vi "Decoratorn2_Main.vi"() -> ()   [LabVIEW 2020]
uses:
  Circle_class/Circle.lvclass
  C:/Projects/DesignPatterns/Decorator2/Object_interface/Object.lvclass
  HappyDecorator_class/HappyDecorator.lvclass
panel:
  in  "Add Decoration?":bool
  out "2D Picture":picture
  # "Run it first without \"Add Decoration?\"\nAnd then with :-)"
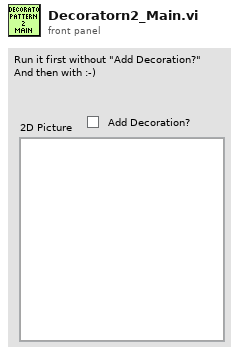
[diagram p1: front panel]
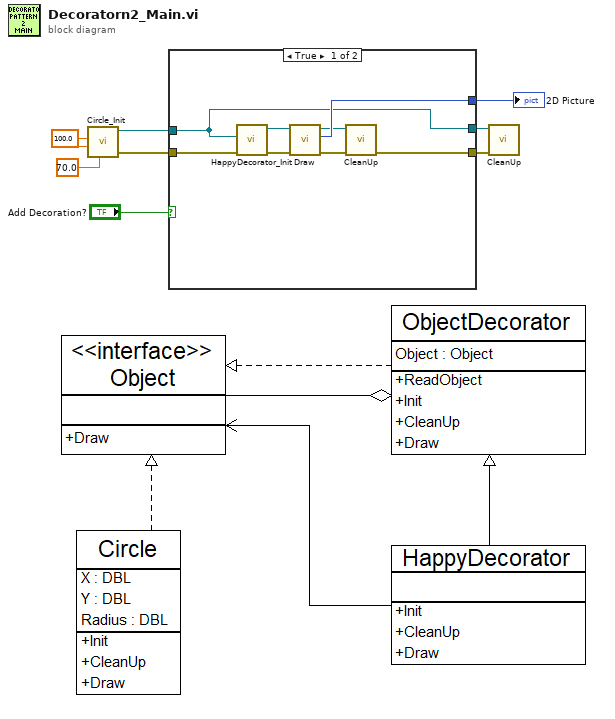
[diagram p0: block diagram]
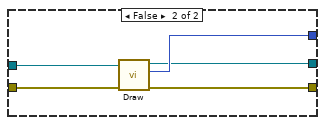
[diagram p2: hidden frame]
diagram:
  w5 = 100.0 ("X")
  n1 = call "Circle_Init.vi"("Radius"=70.0, "Y"=w5, "X"=w5) -> ("error out"=w7:errorcluster, "object out"=w8:refnum<class "Circle.lvclass">)  [unwired: 7 in]
  n2 = case shown="True" "Add Decoration?" {
    tunnel: w8 -> [w13 w21]
    tunnel: w7 -> [w16 w20]
    tunnel: [w15 w19] -> w6
    tunnel: [w14 w18] -> w3
    tunnel: [w13 w17] -> w2
    frame True {
      n3 = call "HappyDecorator_Init.vi"("error in (no error)"=w16, "Object"=w13) -> ("error out"=w12:errorcluster, "object out"=w11:refnum<class "HappyDecorator.lvclass">)  [unwired: 8 in]
      n4 = call-dynamic "Draw.vi"("Error In"=w12, "object in"=w11) -> ("Error Out"=w10:errorcluster, "PictureOut"=w15:picture, "object out"=w9:refnum<class "HappyDecorator.lvclass">)  [unwired: 7 in]
      n5 = call-dynamic "CleanUp.vi"("error in (no error)"=w10, "Object in"=w9) -> ("error out"=w14:errorcluster)  [unwired: 8 in, 1 out]
    }
    frame False {
      n6 = call-dynamic "Draw.vi"("Error In"=w20, "object in"=w21) -> ("Error Out"=w18:errorcluster, "PictureOut"=w19:picture, "object out"=w17:refnum<class "Circle.lvclass">)  [unwired: 7 in]
    }
  }
  "2D Picture" <- w6
  n7 = call-dynamic "CleanUp.vi"("error in (no error)"=w3, "object in"=w2) -> ()  [unwired: 8 in, 2 out]
